vi "Dialog_ShowHideGroups.vi"(8 "error in (no error)":errorcluster, 9 "Table CtlRef In":refnum<vi>, 11 "GroupCol Index":i32=3) -> (0 "error out":errorcluster, 1 "Table CtlRef Out":refnum<vi>)   [LabVIEW 2013]
doc: "Present user with a group selection dialog. Upon clicking Done, un-checked groups will be hidden (row height set to zero)."
uses:
  <vilib>/Utility/miscctls.llb/LVRowAndColumnTypeDef.ctl
  Globals/StdRowHeightGlobal.vi
panel:
  out "item?":bool
  out "In Bounds?":bool
  out "Row":i32
  in  "Cancel":bool
  in  "Done":bool
  in  "Groups Listbox":i32[](listbox) caption="Select groups to SHOW (if checked):"
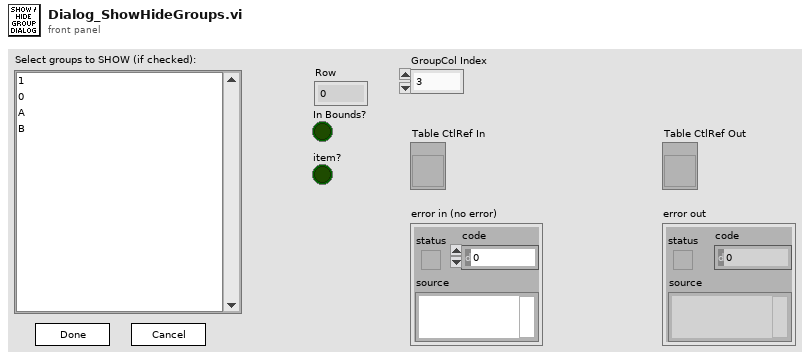
[diagram p1: front panel]
types:
  T1 = typedef "LVRowAndColumnTypeDef.ctl" = cluster{"Row":i32, "Column":i32}
  T2 = typedef "LVPoint32TypeDef.ctl" = cluster{"Horizontal":i32, "Vertical":i32}
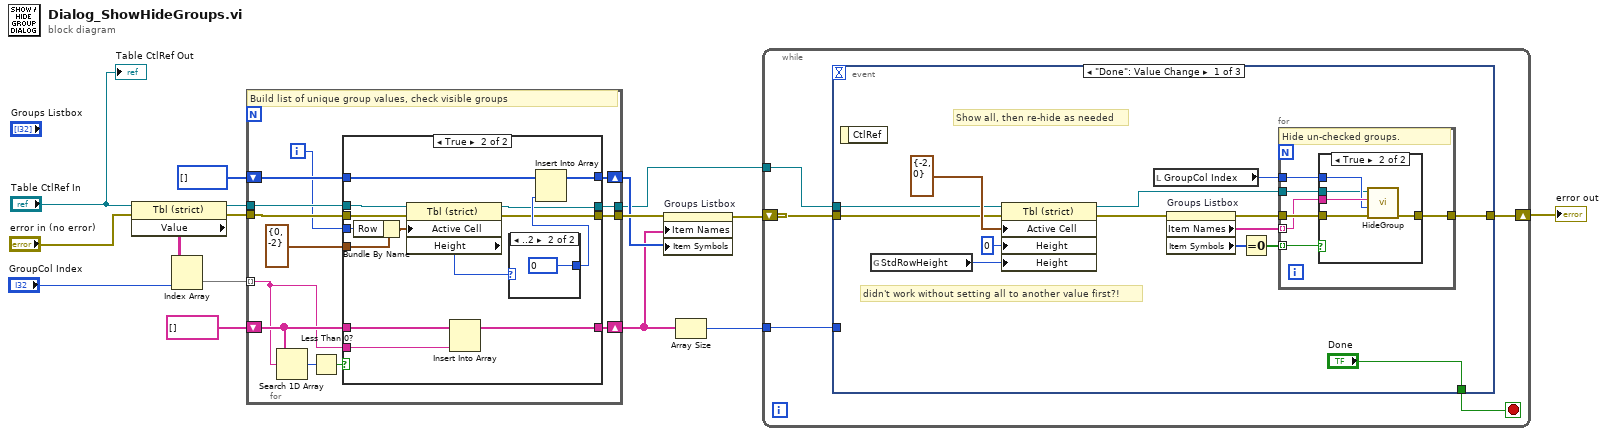
[diagram p0: block diagram]
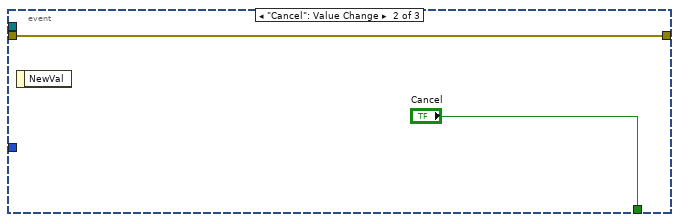
[diagram p3: hidden frame]
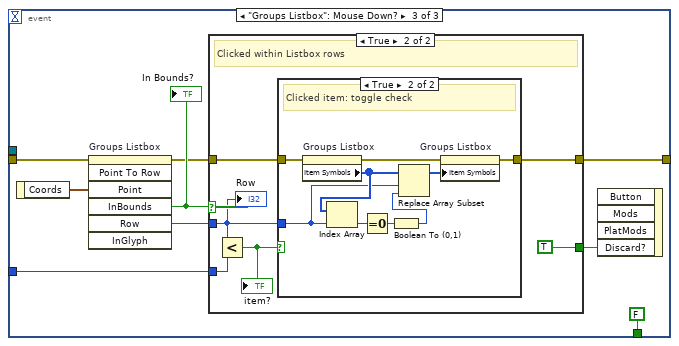
[diagram p4: hidden frame]
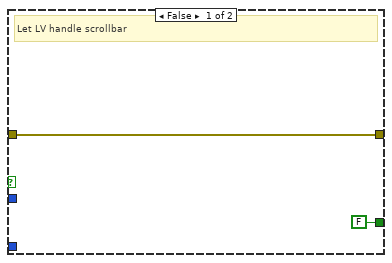
[diagram p5: hidden frame]
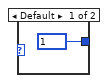
[diagram p8: hidden frame]
diagram:
  n1 = property class="Tbl (strict)"(reference="Table CtlRef In", error in="error in (no error)") -> (reference out=w8:refnum<vi>, error out=w7:errorcluster, "Value"=w15:string[][])
  n2 = Index Array(array=w15, index (col)="GroupCol Index") -> (element=w13:string[])  [unwired: 1 in]
  n3 = for {
    tunnel: w13 -> [w27] mode=indexing
    shift-right: [w28] -> w3
    shift-left: string[] [] ("Item Names") -> [w29]
    tunnel: w8 -> [w22]
    tunnel: w7 -> [w21]
    shift-right: [w23] -> w4
    shift-left: i32[] [] ("Item Symbols") -> [w24]
    tunnel: [w20] -> w5
    tunnel: [w19] -> w1
    i -> [w17]
    # "Build list of unique group values, check visible groups"
    n4 = Search 1D Array(1D array=w29, element=w27) -> (index of element=w25:i32)  [unwired: 1 in]
    n5 = Less Than 0?(x=w25) -> (x < 0?=w26:bool)
    n6 = case shown="True" w26 {
      tunnel: w29 -> [w33 w47]
      tunnel: [w33 w46] -> w28
      tunnel: w27 -> [_ w45]
      tunnel: [w32 w41] -> w23
      tunnel: w24 -> [w32 w42]
      tunnel: w22 -> [w31 w44]
      tunnel: w21 -> [w30 w43]
      tunnel: [w30 w38] -> w20
      tunnel: [w31 w37] -> w19
      tunnel: T1 {"Row"=0, "Column"=-2} ("Active Cell:Active Cell") -> [_ w36]
      tunnel: w17 -> [_ w34]
      frame False {
      }
      frame True {
        n7 = Bundle By Name(cluster=w36, "Row"=w34) -> (w35:T1)
        n8 = property class="Tbl (strict)"(reference=w44, error in=w43, "Active Cell"=w35) -> (reference out=w37:refnum<vi>, error out=w38:errorcluster, "Height"=w39:u32)
        n9 = Insert Into Array(array=w47, new element=w45) -> (w46:string[])  [unwired: 1 in]
        n10 = case shown="..2" w39 {
          tunnel: [1 0] -> w40
          frame Default {
          }
          frame ..2 {
          }
        }
        n11 = Insert Into Array(array=w42, new element=w40) -> (w41:i32[])  [unwired: 1 in]
      }
    }
  }
  n12 = property on="Groups Listbox" class="LstBox (strict)"(error in=w5, "Item Names"=w3, "Item Symbols"=w4) -> (error out=w10:errorcluster)  [unwired: 1 in, 1 out]
  n13 = Array Size(array=w3) -> (size(s)=w2:i32)
  n14 = while {
    shift-right: [w52] -> w11
    shift-left: w10 -> [w53]
    tunnel: w2 -> [w51]
    tunnel: w1 -> [w50]
    stop <- w54 stop-if-true
    n15 = event shown="[0] \"Done\": Value Change" {
      selector: _ -> [_ _ _]
      dyn-events: _ -> [_ _ _]
      timeout: _ -> [_ _ _]
      tunnel: ["Done" "Cancel" FALSE ("Cancel")] -> w54
      tunnel: w53 -> [w58 w82 w91]
      tunnel: [w55 w82 w84] -> w52
      tunnel: w51 -> [_ _ w86]
      tunnel: w50 -> [w57 _ _]
      event "Done": Value Change {
        # "didn't work without setting all to another value first?!"
        # "Show all, then re-hide as needed"
        n16 = event-data() -> ()  [unwired: 1 in, 1 out]
        n17 = global read "StdRowHeightGlobal.vi" "StdRowHeight"() -> (w61:u32)
        n18 = property class="Tbl (strict)"(reference=w57, error in=w58, "Active Cell"=T1 {"Row"=-2, "Column"=0} ("Active Cell:Active Cell"), "Height"=u32 0 ("Active Cell:Cell Size:Height"), "Height"=w61) -> (reference out=w56:refnum<vi>, error out=w59:errorcluster)
        n19 = local read "GroupCol Index"() -> (w63:i32)
        n20 = property on="Groups Listbox" class="LstBox (strict)"(error in=w59) -> (error out=w64:errorcluster, "Item Names"=w67:string[], "Item Symbols"=w66:i32[])  [unwired: 1 in, 1 out]
        n21 = Equal To 0?(x=w66) -> (x = 0?=w65:bool[])
        n22 = for {
          tunnel: w67 -> [w72] mode=indexing
          tunnel: w65 -> [w74] mode=indexing
          tunnel: w64 -> [w73]
          tunnel: w63 -> [w71]
          tunnel: w56 -> [w70]
          tunnel: [w69] -> w55
          # "Hide un-checked groups."
          n23 = case shown="True" w74 {
            tunnel: w73 -> [w75 w80]
            tunnel: w72 -> [_ w79]
            tunnel: w71 -> [_ w78]
            tunnel: w70 -> [_ w77]
            tunnel: [w75 w76] -> w69
            frame False {
            }
            frame True {
              n24 = call "HideGroup.vi"("error in (no error)"=w80, "GroupCol Index"=w78, "String toHide"=w79, "Table CtlRef In"=w77) -> ("error out"=w76:errorcluster)  [unwired: 6 in, 1 out]
            }
          }
        }
      }
      event "Cancel": Value Change {
        n25 = event-data() -> ()  [unwired: 1 in, 1 out]
      }
      event "Groups Listbox": Mouse Down? {
        n26 = event-data() -> ("Coords"=w90:T2)  [unwired: 1 in]
        n27 = invoke on="Groups Listbox" class="LstBox (strict)" method="Point To Row"(error in=w91, "Point"=w90) -> (error out=w85:errorcluster, "InBounds"=w87:bool, "Row"=w89:i32)  [unwired: 5 in, 4 out]
        "In Bounds?" <- w87
        n28 = case shown="True" w87 {
          tunnel: w89 -> [_ w95]
          tunnel: [FALSE ("Discard?") TRUE ("Discard?")] -> w88
          tunnel: w86 -> [_ w98]
          tunnel: w85 -> [w92 w96]
          tunnel: [w92 w94] -> w84
          frame False {
            # "Let LV handle scrollbar"
          }
          frame True {
            # "Clicked within Listbox rows"
            n29 = Less?(x=w95, y=w98) -> (x < y?=w97:bool)
            "item?" <- w97
            n30 = case shown="True" w97 {
              tunnel: w96 -> [w100 w109]
              tunnel: w95 -> [_ w104]
              tunnel: [w100 w106] -> w94
              frame False {
                # "Clicked below items"
              }
              frame True {
                # "Clicked item: toggle check"
                n31 = property on="Groups Listbox" class="LstBox (strict)"(error in=w109) -> (error out=w108:errorcluster, "Item Symbols"=w105:i32[])  [unwired: 1 in, 1 out]
                n32 = Index Array(array=w105, index=w104) -> (element=w102:i32)
                n33 = Equal To 0?(x=w102) -> (x = 0?=w103:bool)
                n34 = Boolean To (0,1)(Boolean=w103) -> (0, 1=w101:i16)
                n35 = Replace Array Subset(array=w105, new element=w101, index=w104) -> (w107:i32[])
                n36 = property on="Groups Listbox" class="LstBox (strict)"(error in=w108, "Item Symbols"=w107) -> (error out=w106:errorcluster)  [unwired: 1 in, 1 out]
              }
            }
            "Row" <- w95
          }
        }
        n37 = event-data("Discard?"=w88) -> ()  [unwired: 4 in, 1 out]
      }
    }
  }
  "error out" <- w11
  "Table CtlRef Out" <- "Table CtlRef In"
